vi "Log Entry Template.vi"(0 "Data In":T2, 11 "Console Entry":string, 14 "Error In":errorcluster) -> (4 "Data Out":T2, 15 "Console log out":string)   [LabVIEW 2019]
doc: "Unpacks a log, and inserts new entry to the log."
uses:
  Controls/Data.ctl
  <vilib>/Utility/error.llb/DialogType.ctl
  <vilib>/Utility/miscctls.llb/LVPointTypeDef.ctl
  Controls/Log_Timeformat.ctl
panel:
  out "Control Tab":T1(tab)
  out "Timestamp":string
  out "Console log in":string
  out "Error Out":errorcluster
  out "Error Message":string
  out "VI-filename":string
  out "Revision Number":u32
  out "VI Description":string
  out "Callers' Names":string[](array[string])
  out "Code Size":u32
  out "VI Type":T3(ring)
  out "Project name":string
  out "Project filepath":path
  out "VI filepath":path
  out "Project Description":string
  out "VI-Name":string
  # "Common Errors:"
  # "0:"
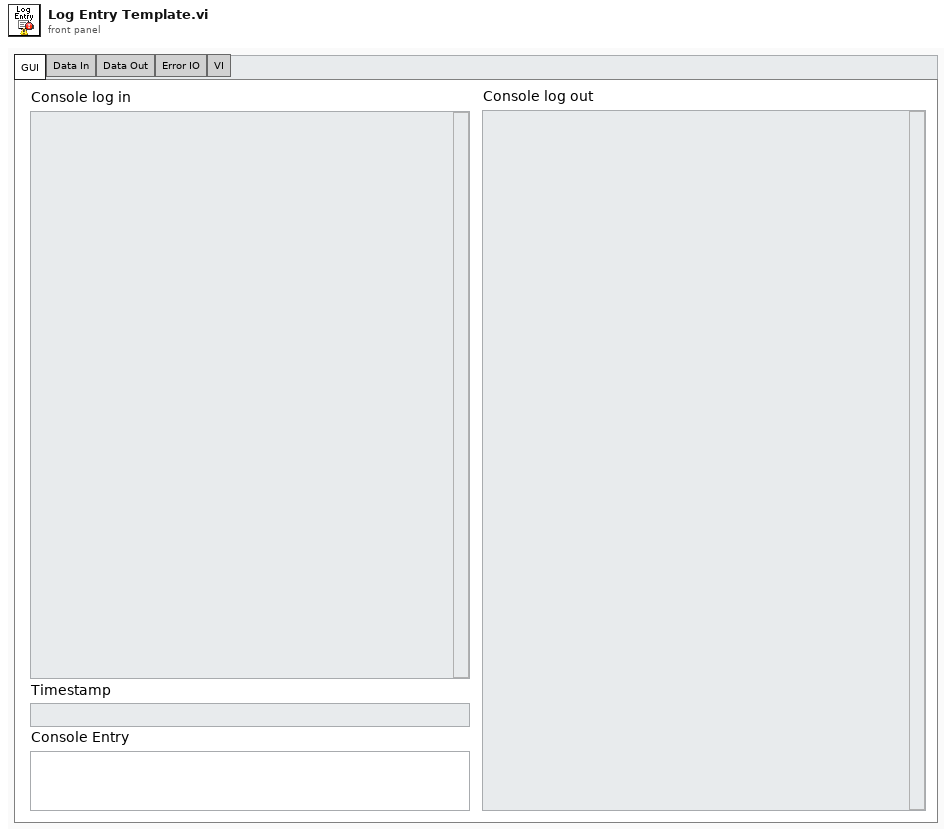
[diagram p1: front panel]
types:
  T1 = enum32{"GUI", "Data In", "Data Out", "Error IO", "VI"}
  T2 = typedef "Data.ctl" = cluster{"Log":string}
  T3 = enum32{"invalid VI type", "Standard VI", "Control VI", "Global VI", "Polymorphic VI", "Configuration VI", "SubSystem", "Facade VI", "Method VI", "Statechart Diagram VI"}
  T4 = typedef "Log_Timeformat.ctl" = string
  T5 = typedef "LVPointTypeDef.ctl" = cluster{"Horizontal":i16, "Vertical":i16}
  T6 = typedef "DialogType.ctl" = u16
  T7 = typedef "LVRectTypeDef.ctl" = cluster{"Left":i16, "Top":i16, "Right":i16, "Bottom":i16}
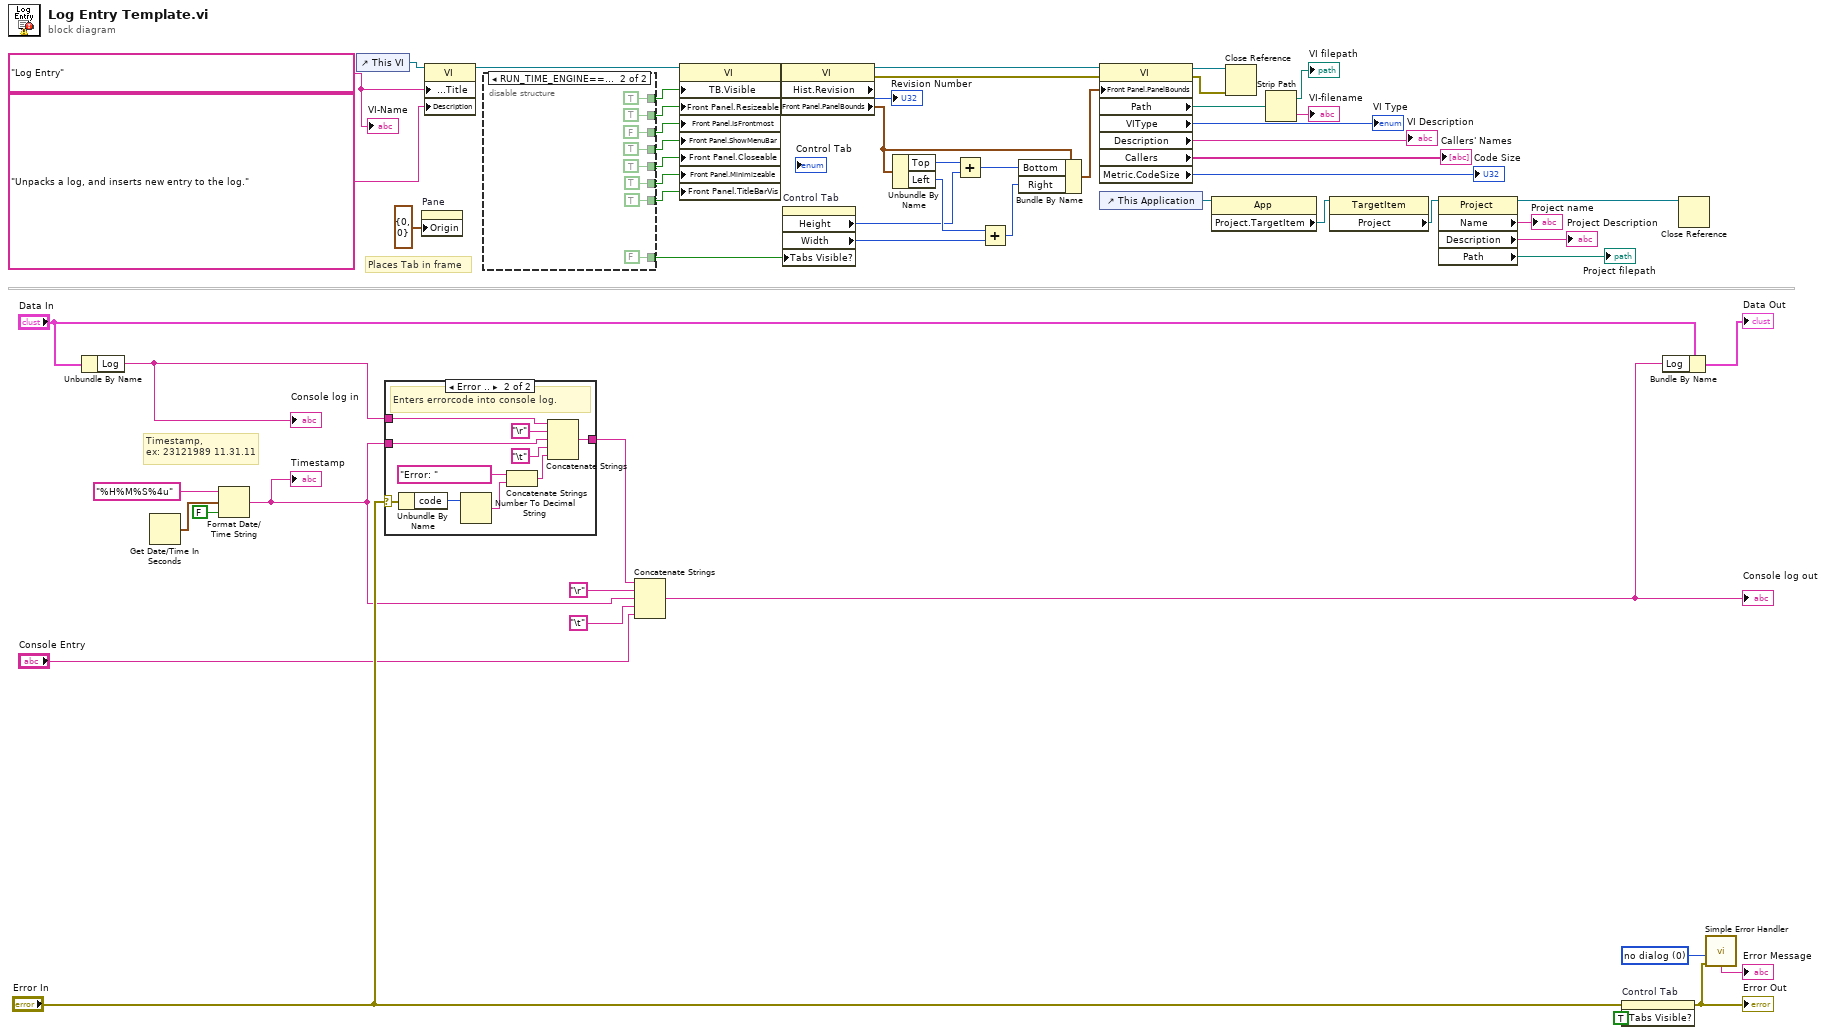
[diagram p0: block diagram]
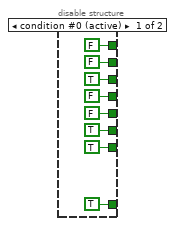
[diagram p3: hidden frame]
diagram:
  w28 = "Log Entry"
  w56 = T6 0 items=["no dialog", "OK message", "continue or stop message", "OK message + warnings", "continue/stop + warnings"] ("type of dialog (OK msg:1)")
  # "Timestamp, \nex: 23121989 11.31.11"
  # "Places Tab in frame"
  n1 = Unbundle By Name("Data In") -> ("Log"=w10:string)
  "Console log in" <- w10
  n2 = Get Date/Time In Seconds() -> (seconds since 1Jan1904=w11:timestamp)
  n3 = Format Date/Time String(time format string (%c)=T4 "%H%M%S%4u", seconds (now)=w11, UTC format=FALSE) -> (date/time string=w5:string)
  "Timestamp" <- w5
  n4 = control-ref of="This VI"() -> (w40:refnum<vi>)
  n5 = case shown="Error .." "Error In" {
    selector: "Error In" -> [_ w62]
    tunnel: w10 -> [w60 w61]
    tunnel: w5 -> [_ w65]
    tunnel: [w60 w63] -> w6
    frame No Error {
    }
    frame Error {
      # "Enters errorcode into console log."
      n6 = Unbundle By Name(w62) -> ("code"=w70:i32)
      n7 = Number To Decimal String(number=w70) -> (decimal integer string=w69:string)  [unwired: 1 in]
      n8 = Concatenate Strings("Error: " ("string"), w69) -> (w68:string)
      n9 = Concatenate Strings(w61, "\r", w65, "\t", w68) -> (w63:string)
    }
  }
  n10 = property on="Pane" class="Pane"("Origin"=T5 {"Horizontal"=0, "Vertical"=0}) -> ()  [unwired: 2 in, 2 out]
  n11 = property class="VI"(reference=w40, "Front Panel.Title"=w28, "Description"="Unpacks a log, and inserts new entry to the log.") -> (reference out=w30:refnum<vi>)  [unwired: 1 in, 1 out]
  n12 = disable-structure "Exe vs Sim" shown="RUN_TIME_ENGINE==True" {
    disable-tunnel: [FALSE ("Tool Bar:Visible") TRUE ("Tool Bar:Visible")] -> w39
    disable-tunnel: [FALSE ("Front Panel Window:Resizable") TRUE ("Front Panel Window:Resizable")] -> w38
    disable-tunnel: [TRUE ("Front Panel Window:Is Frontmost") FALSE ("Front Panel Window:Is Frontmost")] -> w37
    disable-tunnel: [FALSE ("Front Panel Window:Show Menu Bar") TRUE ("Front Panel Window:Show Menu Bar")] -> w36
    disable-tunnel: [FALSE ("Front Panel Window:Closeable") TRUE ("Front Panel Window:Closeable")] -> w35
    disable-tunnel: [TRUE ("Front Panel Window:Title Bar Visible") TRUE ("Front Panel Window:Title Bar Visible")] -> w34
    disable-tunnel: [TRUE ("Front Panel Window:Minimizable") TRUE ("Front Panel Window:Minimizable")] -> w33
    disable-tunnel: [TRUE FALSE] -> w29
    frame condition #0 (active) {
    }
    frame condition #1 {
    }
  }
  n13 = Concatenate Strings(w6, "\r", w5, "\t", "Console Entry") -> (w1:string)
  "Console log out" <- w1
  n14 = property class="VI"(reference=w30, "TB.Visible"=w39, "Front Panel.Resizeable"=w38, "Front Panel.IsFrontmost"=w37, "Front Panel.ShowMenuBar"=w36, "Front Panel.Closeable"=w35, "Front Panel.Minimizeable"=w33, "Front Panel.TitleBarVis"=w34) -> (reference out=w32:refnum<vi>, error out=w31:errorcluster)  [unwired: 1 in]
  n15 = property class="VI"(reference=w32, error in=w31) -> (reference out=w46:refnum<vi>, error out=w42:errorcluster, "Hist.Revision"=→"Revision Number":u32, "Front Panel.PanelBounds"=w47:T7)
  n16 = property on="Control Tab" class="TabCtl (strict)"("Tabs Visible?"=w29) -> ("Height"=w49:u32, "Width"=w53:u32)  [unwired: 2 in, 2 out]
  n17 = Unbundle By Name(w47) -> ("Top"=w48:i16, "Left"=w52:i16)
  n18 = Add(x=w48, y=w49) -> (x+y=w50:u32)
  n19 = Add(x=w52, y=w53) -> (x+y=w51:u32)
  n20 = Bundle By Name(cluster=w47, "Bottom"=w50, "Right"=w51) -> (w45:T7)
  n21 = property on="Window size" class="VI"(reference=w46, error in=w42, "Front Panel.PanelBounds"=w45) -> (reference out=w54:refnum<vi>, error out=w43:errorcluster, "Path"=w27:path, "VIType"=→"VI Type":T3, "Description"=→"VI Description":string, "Callers"=→"Callers' Names":string[], "Metric.CodeSize"=→"Code Size":u32)
  n22 = control-ref of="This Application"() -> (w17:refnum<vi>)
  n23 = property class="App"(reference=w17) -> ("Project.TargetItem"=w22:refnum<vi>)  [unwired: 1 in, 2 out]
  n24 = Close Reference(reference=w54, error in (no error)=w43) -> ()  [unwired: 1 out]
  n25 = Strip Path(path=w27) -> (stripped path=→"VI filepath":path, name=→"VI-filename":string)
  n26 = property class="TargetItem"(reference=w22) -> ("Project"=w21:refnum<vi>)  [unwired: 1 in, 2 out]
  n27 = property class="Project"(reference=w21) -> (reference out=w15:refnum<vi>, "Name"=→"Project name":string, "Description"=→"Project Description":string, "Path"=→"Project filepath":path)  [unwired: 1 in, 1 out]
  n28 = property on="Control Tab" class="TabCtl (strict)"(error in="Error In", "Tabs Visible?"=TRUE) -> (error out=w14:errorcluster)  [unwired: 1 in, 1 out]
  "Error Out" <- w14
  n29 = Bundle By Name(cluster="Data In", "Log"=w1) -> (→"Data Out":T2)
  n30 = Close Reference(reference=w15) -> ()  [unwired: 1 in, 1 out]
  n31 = call <vilib>:"Simple Error Handler.vi"("type of dialog (OK msg:1)"=w56, "error in (no error)"=w14) -> ("message"=→"Error Message":string)  [unwired: 3 in, 4 out]
  "VI-Name" <- w28
